vi "getILCMap.vi"(11 "ILCCommunications in":refnum<class "ILCCommunications.lvclass">) -> (2 "ILCMap":T1[][](array[typedef]), 3 "ILCCommunications out":refnum<class "ILCCommunications.lvclass">)   [LabVIEW 2016, in "ILCCommunications.lvclass"]
uses:
  ILCCommunications.lvclass
  Types/ILCMap.ctl
  Types/ILCTypes.ctl
  ILCCommunications.lvclass/ILCCommunications.ctl
  Types/M1M3SupportTypes.lvlib
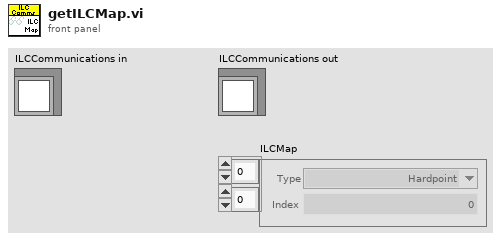
[diagram p1: front panel]
types:
  T1 = typedef "M1M3SupportTypes.lvlib/ILCMap.ctl" = cluster{"Index":i32, "Type":T2}
  T2 = typedef "M1M3SupportTypes.lvlib/ILCTypes.ctl" = enum16{"Hardpoint", "Force"}
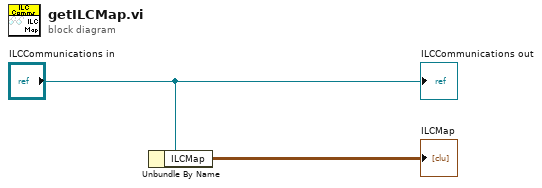
[diagram p0: block diagram]
diagram:
  n1 = Unbundle By Name("ILCCommunications in") -> ("ILCMap"=→"ILCMap":T1[][])
  "ILCCommunications out" <- "ILCCommunications in"
